vi "Panel Resized.vi"(6 "Sizing Refnums":T2, 8 "error in (no error)":errorcluster, 9 "Origin":cluster{"H":i16, "V":i16}, 10 "NewBnds":T1, 11 "Size Constraints":cluster{"min tab width":i32, "w/h":dbl}) -> (0 "error out":errorcluster)   [LabVIEW 2025]
uses:
  <vilib>/Utility/miscctls.llb/LVRectTypeDef.ctl
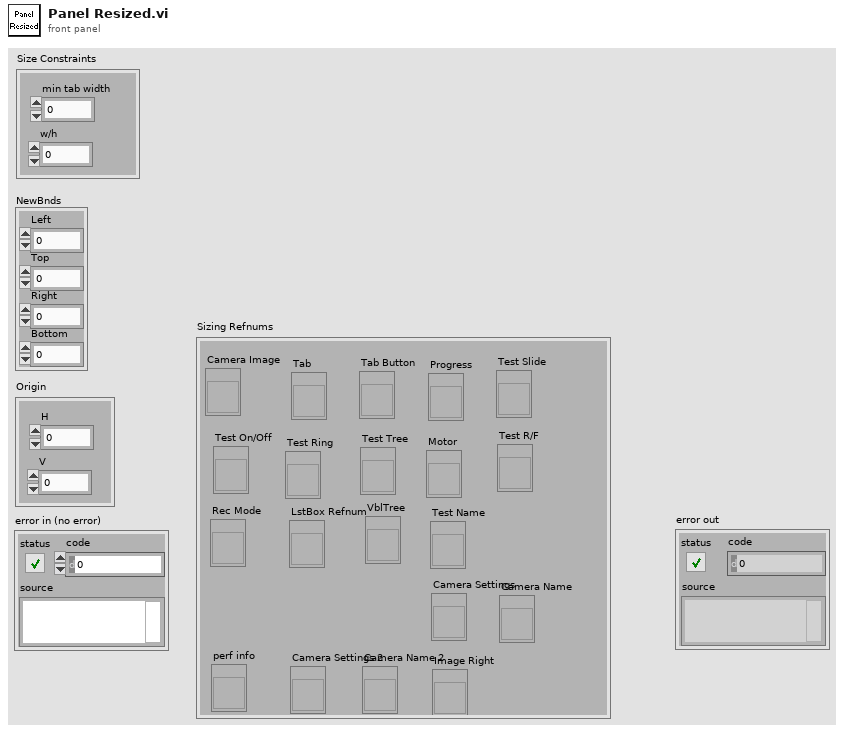
[diagram p1: front panel]
types:
  T1 = typedef "LVRectTypeDef.ctl" = cluster{"Left":i16, "Top":i16, "Right":i16, "Bottom":i16}
  T2 = cluster{"Camera Image":refnum<vi>, "Tab":refnum<vi>, "Tab Button":refnum<vi>, "Rec Mode":refnum<vi>, "Test Slide":refnum<vi>, "Test On/Off":refnum<vi>, "Test Ring":refnum<vi>, "Test R/F":refnum<vi>, "Test Name":refnum<vi>, "Motor":refnum<vi>, "Progress":refnum<vi>, "LstBox Refnum":refnum<vi>, "Test Tree":refnum<vi>, "VblTree":refnum<vi>, "Camera Settings":refnum<vi>, "Camera Name":refnum<vi>, "perf info":refnum<vi>, "Camera Settings 2":refnum<vi>, "Camera Name 2":refnum<vi>, "Image Right":refnum<vi>}
  T3 = typedef "LVPositionTypeDef.ctl" = cluster{"Left":i32, "Top":i32}
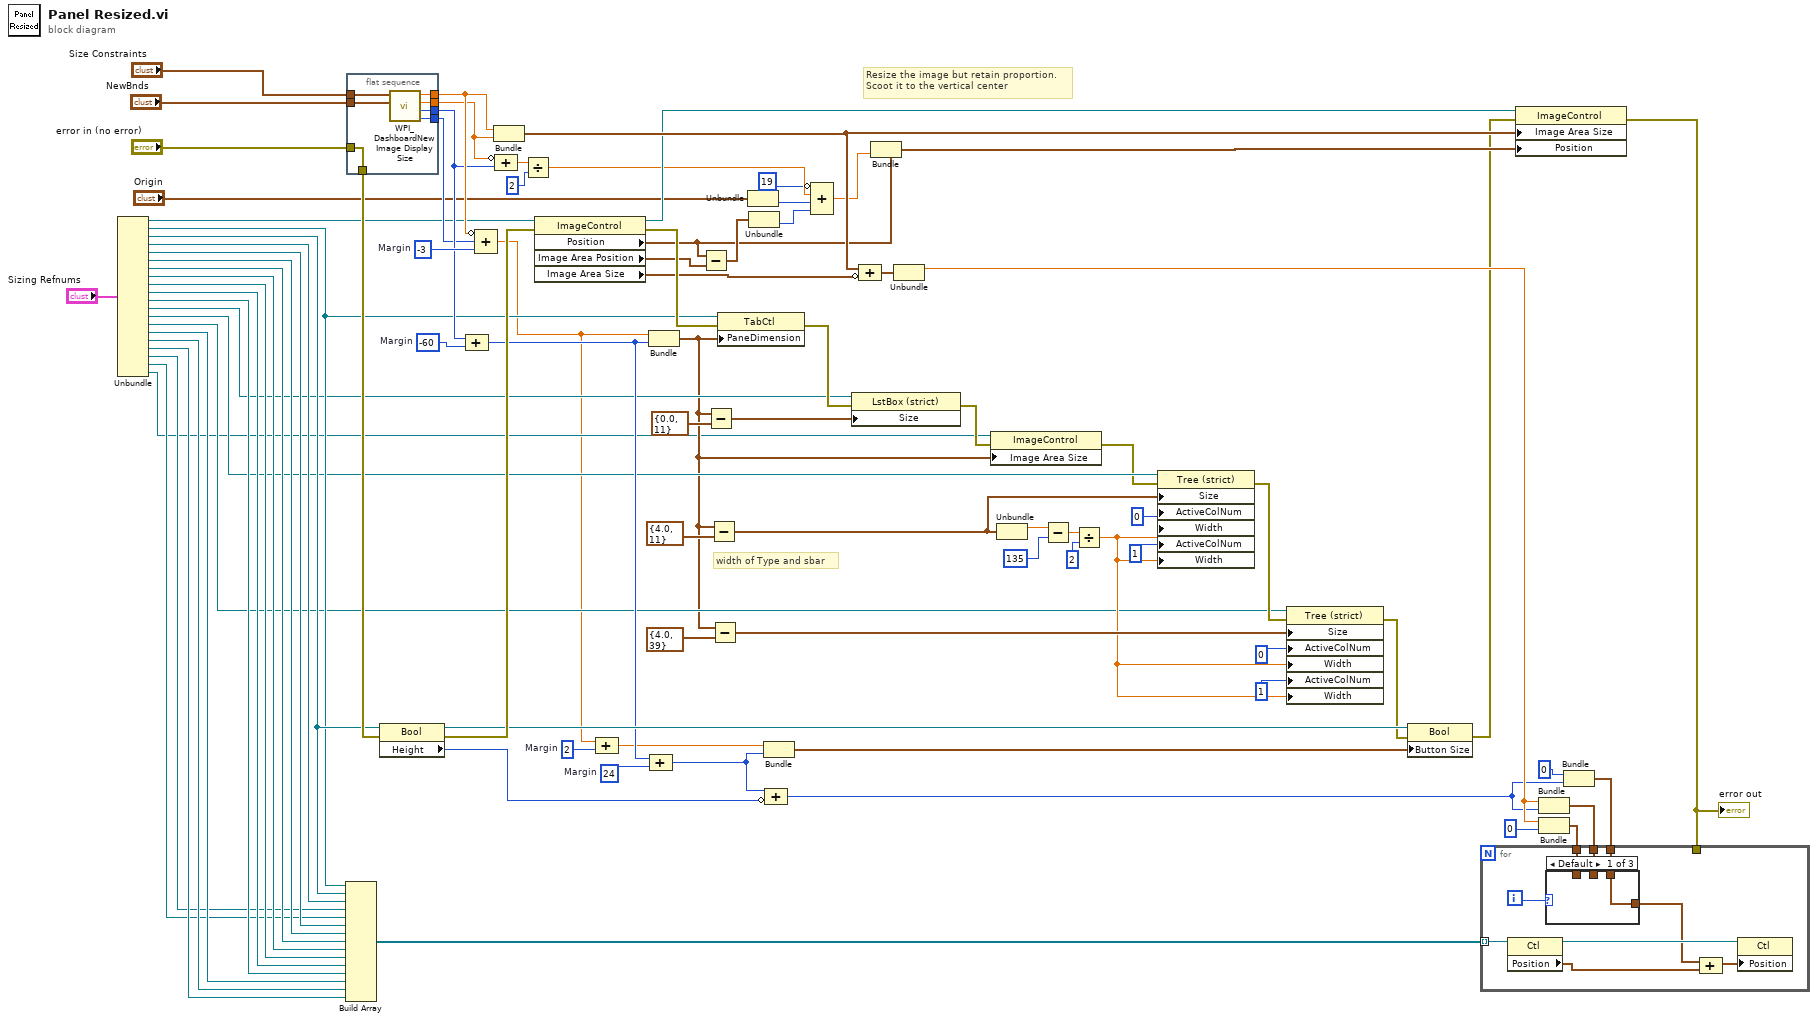
[diagram p0: block diagram]
diagram:
  w76 = 24  # Margin
  w74 = 2  # Margin
  w71 = -60  # Margin
  w80 = -3  # Margin
  # "width of Type and sbar"
  # "Resize the image but retain proportion.\nScoot it to the vertical center"
  n1 = Unbundle("Sizing Refnums") -> ("Camera Image"=w45:refnum<vi>, "Tab"=w46:refnum<vi>, "Tab Button"=w54:refnum<vi>, "Rec Mode"=w22:refnum<vi>, "Test Slide"=w21:refnum<vi>, "Test On/Off"=w20:refnum<vi>, "Test Ring"=w19:refnum<vi>, "Test R/F"=w18:refnum<vi>, "Test Name"=w17:refnum<vi>, "Motor"=w16:refnum<vi>, "Progress"=w15:refnum<vi>, "LstBox Refnum"=w14:refnum<vi>, "Test Tree"=w13:refnum<vi>, "VblTree"=w12:refnum<vi>, "Camera Settings"=w9:refnum<vi>, "Camera Name"=w8:refnum<vi>, "perf info"=w7:refnum<vi>, "Camera Settings 2"=w6:refnum<vi>, "Camera Name 2"=w5:refnum<vi>, "Image Right"=w2:refnum<vi>)
  n2 = Build Array(w46, w54, w22, w6, w5, w21, w20, w19, w18, w17, w16, w15, w9, w8, w7) -> (w89:refnum<vi>[])
  n3 = flat-sequence {
    tunnel: "NewBnds" -> [w96]
    tunnel: "Size Constraints" -> [w95]
    tunnel: [w94] -> w70
    tunnel: [w93] -> w77
    tunnel: [w92] -> w78
    tunnel: [w91] -> w79
    tunnel: [w90] -> w88
    tunnel: "error in (no error)" -> [w90]
    frame #0 {
      n4 = call <vilib>:"WPI_DashboardNew Image Display Size.vi"("NewBnds"=w96, "Size Constraints"=w95) -> ("Window Width"=w94:i16, "Window Height"=w92:i16, "Height"=w93:dbl, "Width"=w91:dbl)  [unwired: 6 in]
    }
  }
  n5 = property class="Bool"(reference=w54, error in=w88) -> (reference out=w83:refnum<vi>, error out=w87:errorcluster, "Height"=w82:u32)
  n6 = Compound Arithmetic op=unknown(w78, w71) -> (w75:i32)
  n7 = Compound Arithmetic op=ADD(invert w79, w70, w80) -> (w1:dbl)
  n8 = Bundle("Width"=w79, "Height"=w77) -> (w66:cluster{"Width":dbl, "Height":dbl})  [unwired: 1 in]
  n9 = Compound Arithmetic op=ADD(invert w77, w78) -> (w58:dbl)
  n10 = Divide(x=w58, y=2) -> (x/y=w60:dbl)
  n11 = property class="ImageControl"(reference=w45, error in=w87) -> (reference out=w63:refnum<vi>, error out=w86:errorcluster, "Position"=w62:T3, "Image Area Position"=w57:cluster{"Left":i32, "Top":i32}, "Image Area Size"=w68:cluster{"Width":u32, "Height":u32})
  n12 = Compound Arithmetic op=ADD(w1, w74) -> (w73:dbl)
  n13 = Bundle(w1, w75) -> (w11:cluster{dbl, i32})  [unwired: 1 in]
  n14 = Compound Arithmetic op=ADD(w75, w76) -> (w81:i32)
  n15 = Subtract(x=w62, y=w57) -> (x-y=w64:T3)
  n16 = Subtract(x=w11, y=cluster{dbl, i32} {0.0, 11}) -> (x-y=w43:cluster{dbl, i32})
  n17 = Subtract(x=w11, y=cluster{dbl, i32} {4.0, 11}) -> (x-y=w34:cluster{dbl, i32})
  n18 = Subtract(x=w11, y=cluster{dbl, i32} {4.0, 39}) -> (x-y=w39:cluster{dbl, i32})
  n19 = property class="TabCtl"(reference=w46, error in=w86, "PaneDimension"=w11) -> (error out=w44:errorcluster)  [unwired: 1 out]
  n20 = Unbundle("Origin") -> ("V"=w51:i16)  [unwired: 1 out]
  n21 = Unbundle(w64) -> ("Top"=w65:i32)  [unwired: 1 out]
  n22 = Bundle(w73, w81) -> (w72:cluster{dbl, i32})  [unwired: 1 in]
  n23 = Compound Arithmetic op=ADD(w81, invert w82) -> (w25:u32)
  n24 = Compound Arithmetic op=ADD(invert 19, w60, w51, w65) -> (w61:dbl)
  n25 = property class="LstBox (strict)"(reference=w14, error in=w44, "Size"=w43) -> (error out=w10:errorcluster)  [unwired: 1 out]
  n26 = Compound Arithmetic op=ADD(w66, invert w68) -> (w69:cluster{"Width":dbl, "Height":dbl})
  n27 = Bundle(cluster=w62, "Top"=w61) -> (w67:T3)  [unwired: 1 in]
  n28 = Unbundle(w69) -> ("Width"=w84:dbl)  [unwired: 1 out]
  n29 = property class="ImageControl"(reference=w2, error in=w10, "Image Area Size"=w11) -> (error out=w3:errorcluster)  [unwired: 1 out]
  n30 = Unbundle(w34) -> (w33:dbl)  [unwired: 1 out]
  n31 = Subtract(x=w33, y=135 ("Active Cell:Active Column Number")) -> (x-y=w29:dbl)
  n32 = Divide(x=w29, y=2 ("Active Cell:Active Column Number")) -> (x/y=w24:dbl)
  n33 = property class="Tree (strict)"(reference=w13, error in=w3, "Size"=w34, "ActiveColNum"=0 ("Active Cell:Active Column Number"), "Width"=w24, "ActiveColNum"=1 ("Active Cell:Active Column Number"), "Width"=w24) -> (error out=w38:errorcluster)  [unwired: 1 out]
  n34 = property class="Tree (strict)"(reference=w12, error in=w38, "Size"=w39, "ActiveColNum"=0 ("Active Cell:Active Column Number"), "Width"=w24, "ActiveColNum"=1 ("Active Cell:Active Column Number"), "Width"=w24) -> (error out=w37:errorcluster)  [unwired: 1 out]
  n35 = property class="Bool"(reference=w83, error in=w37, "Button Size"=w72) -> (error out=w4:errorcluster)  [unwired: 1 out]
  n36 = property class="ImageControl"(reference=w63, error in=w4, "Image Area Size"=w66, "Position"=w67) -> (error out=w50:errorcluster)  [unwired: 1 out]
  "error out" <- w50
  n37 = Bundle("Width"=w84, w25) -> (w56:cluster{"Width":dbl, u32})  [unwired: 1 in]
  n38 = Bundle("Width"=w84, 0) -> (w55:cluster{"Width":dbl, i32})  [unwired: 1 in]
  n39 = Bundle(0, w25) -> (w26:cluster{i32, u32})  [unwired: 1 in]
  n40 = for {
    tunnel: w89 -> [w105] mode=indexing
    tunnel: w56 -> [w99]
    tunnel: w55 -> [w100]
    tunnel: w50 -> [_]
    tunnel: w26 -> [w98]
    i -> [w101]
    n41 = property class="Ctl"(reference=w105) -> (reference out=w104:refnum<vi>, "Position"=w103:T3)  [unwired: 1 in, 1 out]
    n42 = case shown="Default" w101 {
      tunnel: w100 -> [_ w107 _]
      tunnel: w99 -> [_ _ w108]
      tunnel: w98 -> [w106 _ _]
      tunnel: [w106 w107 w108] -> w97
      frame Default {
      }
      frame 0, 1 {
      }
      frame 2..4 {
      }
    }
    n43 = Compound Arithmetic op=ADD(w97, w103) -> (w102:cluster{dbl, u32})
    n44 = property class="Ctl"(reference=w104, "Position"=w102) -> ()  [unwired: 1 in, 2 out]
  }
